vi "switch.vi"(8 "error in (no error)":errorcluster, 10 "Positive?":bool=TRUE, 11 "Switch port (in)":refnum<visa-resource-name>="COM6") -> (0 "error out":errorcluster, 3 "Switch port (out)":refnum<visa-resource-name>)   [LabVIEW 2017]
uses:
  <vilib>/Instr/_visa.llb/VISA Configure Serial Port (Serial Instr).vi
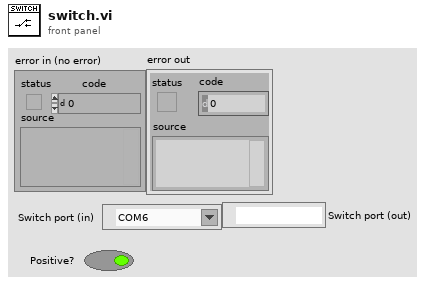
[diagram p1: front panel]
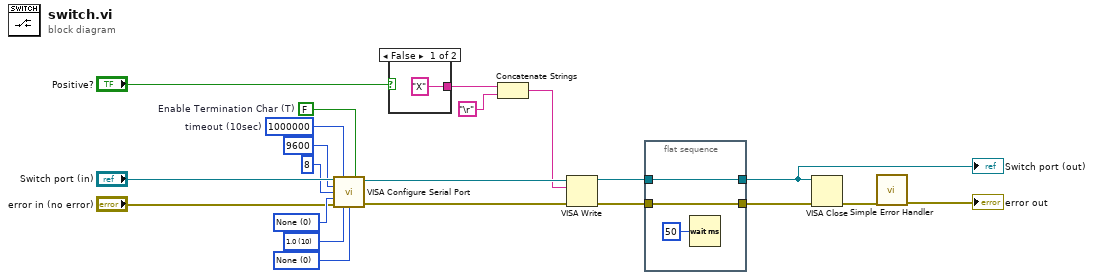
[diagram p0: block diagram]
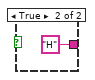
[diagram p2: hidden frame]
diagram:
  w11 = u16 0 items=["None"=0, "XON/XOFF"=1, "RTS/CTS"=2, "DTR/DSR"=4] ("flow control")
  w13 = u16 10 items=["1.0"=10, "1.5"=15, "2.0"=20] ("stop bits")
  w16 = u16 0 items=["None", "Odd", "Even", "Mark", "Space"] ("parity")
  w14 = FALSE  # Enable Termination Char (T)
  w15 = u32 1000000  # timeout (10sec)
  n1 = call-poly "VISA Configure Serial Port"("VISA resource name"="Switch port (in)", "timeout (10sec)"=w15, "Enable Termination\nChar (T)"=w14, "baud rate (9600)"=u32 9600 ("baud rate"), "data bits (8)"=u16 8 ("data bits"), "parity (0:none)"=w16, "error in (no error)"="error in (no error)", "stop bits (10: 1 bit)"=w13, "flow control (0:none)"=w11) -> ("VISA resource name out"=w19:refnum<visa-resource-name>, "error out"=w18:errorcluster)  [unwired: 5 in]
  n2 = case shown="False" "Positive?" {
    tunnel: ["X" ("concatenated string") "H" ("concatenated string")] -> w1
    frame False {
    }
    frame True {
    }
  }
  n3 = Concatenate Strings(w1, "\r") -> (w9:string)
  n4 = VISA Write(VISA resource name=w19, write buffer=w9, error in (no error)=w18) -> (VISA resource name out=w7:refnum<visa-resource-name>, error out=w5:errorcluster)  [unwired: 1 out]
  n5 = flat-sequence {
    tunnel: [w26] -> w8
    tunnel: w7 -> [w26]
    tunnel: [w25] -> w6
    tunnel: w5 -> [w25]
    frame #0 {
      n6 = Wait (ms)(milliseconds to wait=u32 50) -> ()  [unwired: 1 out]
    }
  }
  n7 = VISA Close(VISA resource name=w8, error in (no error)=w6) -> (error out=w20:errorcluster)
  n8 = call <vilib>:"Simple Error Handler.vi"("error in (no error)"=w20) -> ("error out"=→"error out":errorcluster)  [unwired: 4 in, 4 out]
  "Switch port (out)" <- w8
